vi "IdentifyAndReadInstr.vi"(8 "error in (no error)":errorcluster, 11 "VISA Resource Name":refnum<visa-resource-name>) -> (0 "error out":errorcluster, 1 "Instrument":T1=enum."LkShr 340 chA&B", 2 "Identified":bool, 3 "VISA Resource Name Out":refnum<visa-resource-name>)   [LabVIEW 2016]
uses:
  Device/Device type.ctl
  GPIB/VISA  Send Receive.vi
  <vilib>/Utility/error.llb/Error Cluster From Error Code.vi
  <vilib>/ErrorRing/Error Ring.xnode
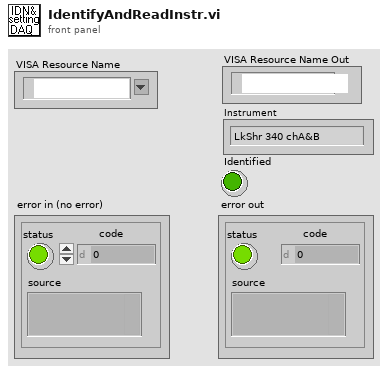
[diagram p1: front panel]
types:
  T1 = typedef "Device type.ctl" = enum16{"NONE", "Neocera 21", "LakeShore 335", "LakeShore 336", "LakeShore 340", "LkShr 340 chA&B", "LakeShore 370", "SRS 850", "SRS 830", "LR 700", "EG&G 5302", "EG&G 7260", "EG&G 7280", "AH 2500", "Keithley meter", "Keithley electrometer", "Keithley 182", "HP 5385", "HP 53181", "HP 53132", "ITC503", "IPS120", "Oxford Mercury IPS", "Oxford PS", "Test", "DC Facility Magnet", "Cryomagnetics PS", "Keithley 2400", "Keithley current source", "Cryo-Con 22C", "HP87NN", "HP4395A"}
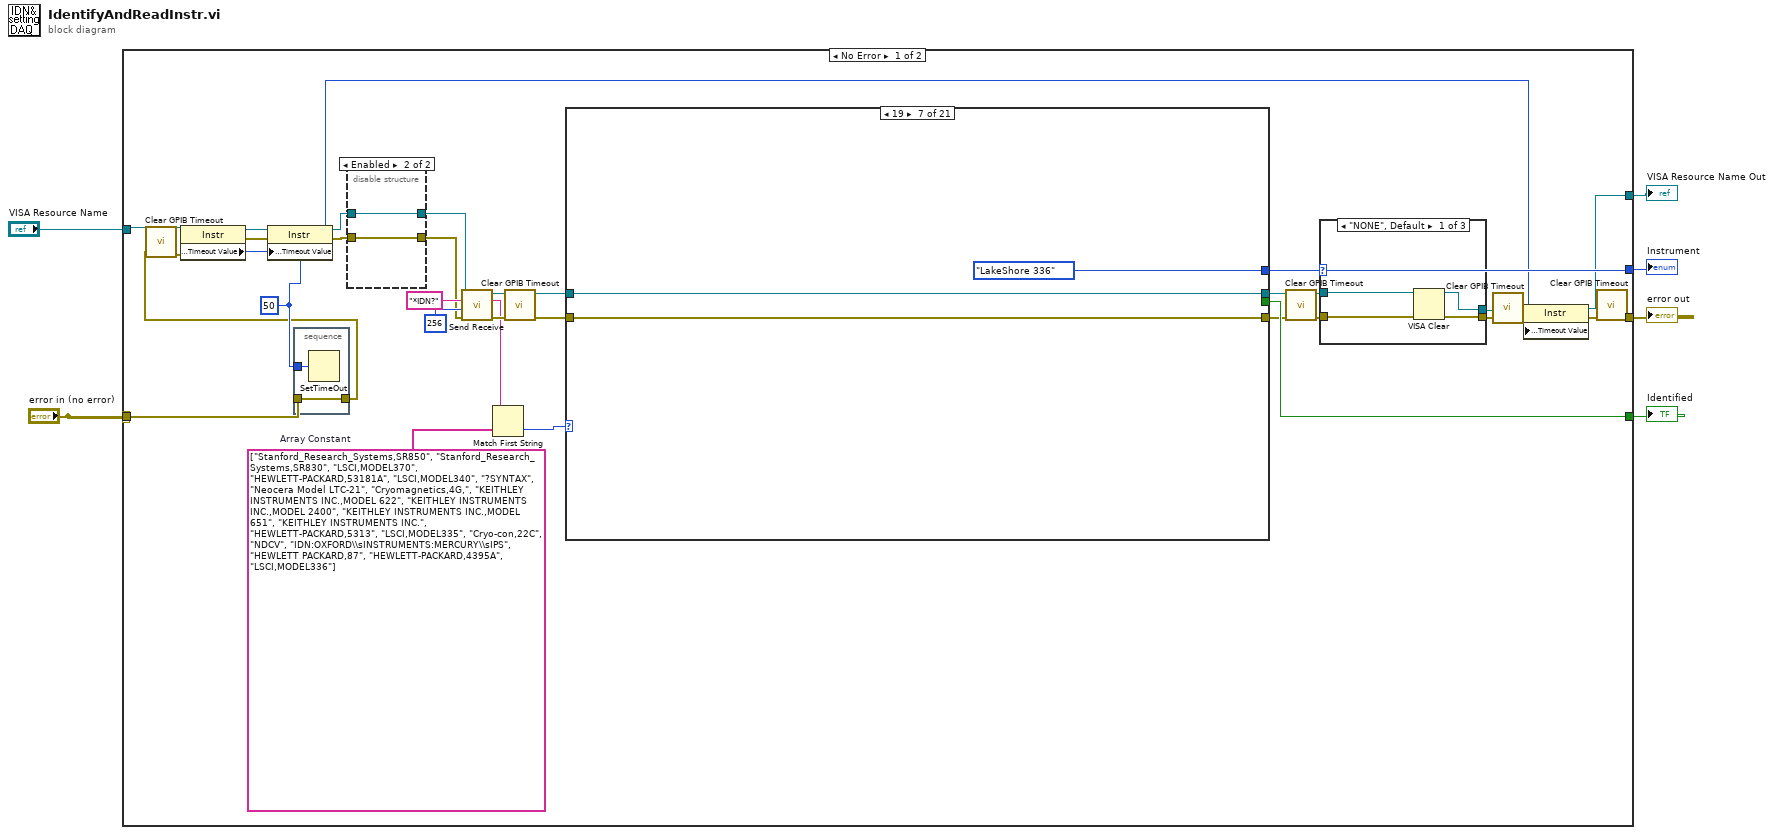
[diagram p0: block diagram]
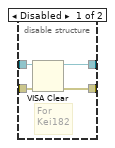
[diagram p2: hidden frame]
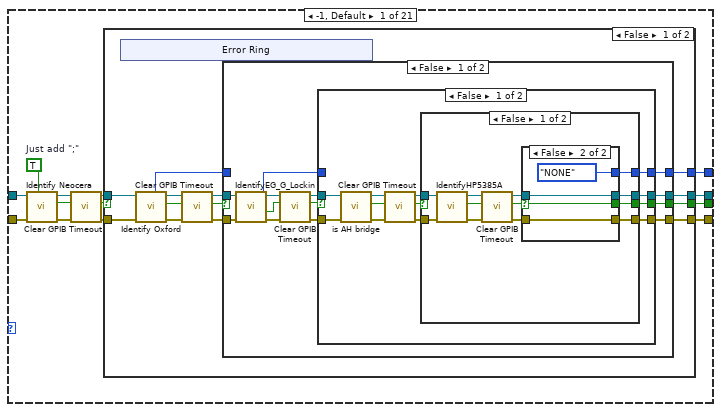
[diagram p5: hidden frame]
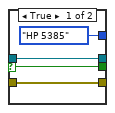
[diagram p6: hidden frame]
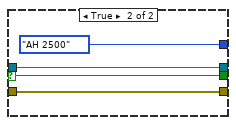
[diagram p7: hidden frame]
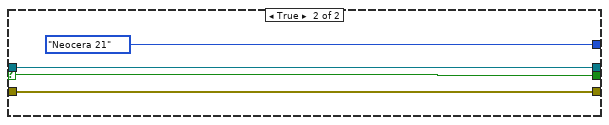
[diagram p10: hidden frame]
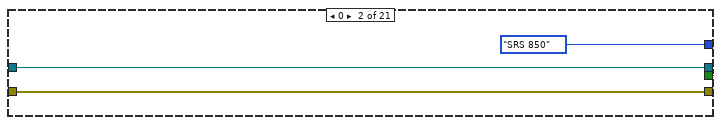
[diagram p11: hidden frame]
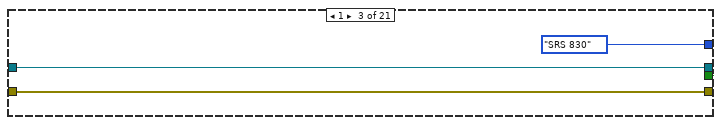
[diagram p12: hidden frame]
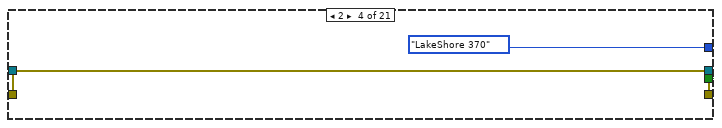
[diagram p13: hidden frame]
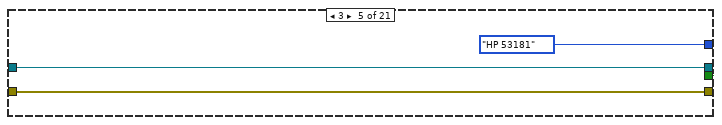
[diagram p14: hidden frame]
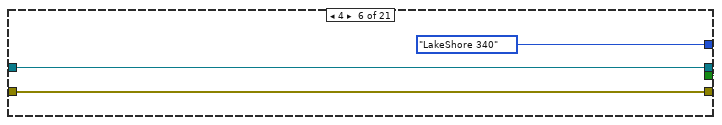
[diagram p15: hidden frame]
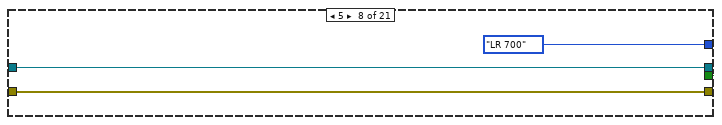
[diagram p16: hidden frame]
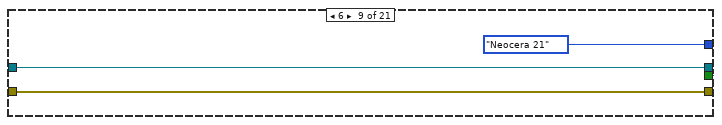
[diagram p17: hidden frame]
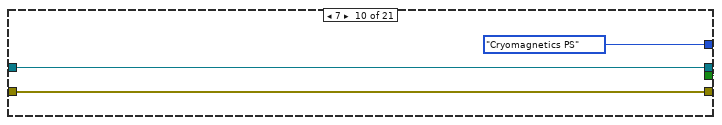
[diagram p18: hidden frame]
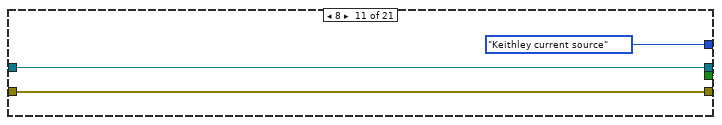
[diagram p19: hidden frame]
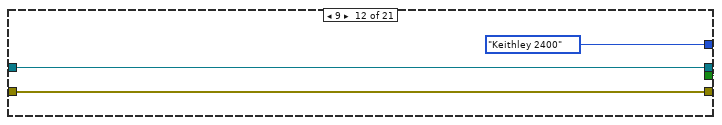
[diagram p20: hidden frame]
diagram:
  n1 = case shown="No Error" "error in (no error)" {
    tunnel: "error in (no error)" -> [w29 w230]
    tunnel: [w8 w230] -> w3
    tunnel: [w32 FALSE ("Identified")] -> w6
    tunnel: [w19 Device_type."NONE" ("Instrument")] -> w1
    tunnel: "VISA Resource Name" -> [w9 w228]
    tunnel: [w7 w228] -> w2
    frame No Error {
      w37 = string[] ["Stanford_Research_Systems,SR850", "Stanford_Research_Systems,SR830", "LSCI,MODEL370", "HEWLETT-PACKARD,53181A", "LSCI,MODEL340", "?SYNTAX", "Neocera Model LTC-21", "Cryomagnetics,4G,", "KEITHLEY INSTRUMENTS INC.,MODEL 622", "KEITHLEY INSTRUMENTS INC.,MODEL 2400", "KEITHLEY INSTRUMENTS INC.,MODEL 651", "KEITHLEY INSTRUMENTS INC.", "HEWLETT-PACKARD,5313", "LSCI,MODEL335", "Cryo-con,22C", "NDCV", "IDN:OXFORD\\sINSTRUMENTS:MERCURY\\sIPS", "HEWLETT PACKARD,87", "HEWLETT-PACKARD,4395A", "LSCI,MODEL336"]  # Array Constant
      w26 = 50 ("new timeout (10000)")
      n2 = stacked-sequence {
        tunnel: w29 -> [w53]
        tunnel: [w53] -> w10
        tunnel: w26 -> [w52]
        frame #0 {
          n3 = SetTimeOut(1:w52) -> ()  [unwired: 1 out]
        }
      }
      n4 = call "Clear GPIB Timeout.vi"("error in (no error)"=w10) -> ("error out"=w17:errorcluster)  [unwired: 1 in, 9 out]
      n5 = property class="Instr"(reference=w9, error in=w17) -> (reference out=w27:refnum<visa-resource-name>, error out=w25:errorcluster, "General Settings:Timeout Value"=w18:u32)
      n6 = property class="Instr"(reference=w27, error in=w25, "General Settings:Timeout Value"=w26) -> (reference out=w13:refnum<visa-resource-name>, error out=w14:errorcluster)
      n7 = disable-structure shown="Enabled" {
        disable-tunnel: w14 -> [w41 w42]
        disable-tunnel: w13 -> [w40 w43]
        disable-tunnel: [w39 w43] -> w12
        disable-tunnel: [w38 w42] -> w11
        frame Disabled {
          # "For\nKei182"
          n8 = VISA Clear(VISA resource name=w40, error in (no error)=w41) -> (VISA resource name out=w39:refnum<visa-resource-name>, error out=w38:errorcluster)
        }
        frame Enabled {
        }
      }
      n9 = call-poly "Send Receive.vi"("error in (no error)"=w11, "Receive count"=256 ("count"), "data string in"="*IDN?" ("data string"), "VISA Resource Name"=w12) -> ("error out"=w34:errorcluster, "data string out"=w33:string, "VISA Resource Name Out"=w28:refnum<visa-resource-name>)  [unwired: 5 in]
      n10 = Match First String(2:w37, 3:w33) -> (0:w36:i32)  [unwired: 1 out]
      n11 = call "Clear GPIB Timeout.vi"("error in (no error)"=w34) -> ("error out"=w31:errorcluster)  [unwired: 1 in, 9 out]
      n12 = case shown="19" w36 {
        tunnel: w31 -> [w63 w137 w141 w145 w149 w153 w157 w161 w165 w169 w173 w177 w183 w188 w192 w196 w200 w203 w215 w219 w223]
        tunnel: [w64 w137 w141 w145 w149 w153 w157 w161 w165 w169 w173 w177 w180 w188 w192 w196 w200 w202 w215 w219 w223] -> w24
        tunnel: [w61 TRUE ("Identified") TRUE ("Identified") TRUE ("Identified") TRUE ("Identified") TRUE ("Identified") TRUE ("Identified") TRUE ("Identified") TRUE ("Identified") TRUE ("Identified") TRUE ("Identified") TRUE ("Identified") TRUE ("Identified") TRUE ("Identified") TRUE ("Identified") TRUE ("Identified") TRUE ("Identified") TRUE ("Identified") TRUE ("Identified") TRUE ("Identified") TRUE ("Identified")] -> w32
        tunnel: [w62 Device_type."SRS 850" ("Instrument") Device_type."SRS 830" ("Instrument") Device_type."LakeShore 370" ("Instrument") Device_type."HP 53181" ("Instrument") Device_type."LakeShore 340" ("Instrument") Device_type."LakeShore 336" ("Instrument") Device_type."LR 700" ("Instrument") Device_type."Neocera 21" ("Instrument") Device_type."Cryomagnetics PS" ("Instrument") Device_type."Keithley current source" ("Instrument") Device_type."Keithley 2400" ("Instrument") Device_type."Keithley electrometer" ("Instrument") Device_type."Keithley meter" ("Instrument") Device_type."HP 53132" ("Instrument") Device_type."LakeShore 335" ("Instrument") Device_type."Cryo-Con 22C" ("Instrument") Device_type."Keithley 182" ("Instrument") Device_type."Oxford Mercury IPS" ("Instrument") Device_type."HP87NN" ("Instrument") Device_type."HP4395A" ("Instrument")] -> w19
        tunnel: w28 -> [w59 w136 w140 w144 w148 w152 w156 w160 w164 w168 w172 w176 w182 w187 w191 w195 w199 w206 w216 w220 w224]
        tunnel: [w60 w136 w140 w144 w148 w152 w156 w160 w164 w168 w172 w176 w179 w187 w191 w195 w199 w204 w216 w220 w224] -> w22
        frame -1, Default {
          w55 = TRUE  # Just add ";"
          n13 = call "Identify Neocera.vi"("Just add \";\""=w55, "error in (no error)"=w63, "VISA Resource Name"=w59) -> ("error out"=w57:errorcluster, "Identified"=w54:bool, "VISA Resource Name Out"=w58:refnum<visa-resource-name>)  [unwired: 6 out]
          n14 = call "Clear GPIB Timeout.vi"("error in (no error)"=w57) -> ("error out"=w56:errorcluster)  [unwired: 1 in, 9 out]
          n15 = case shown="False" w54 {
            selector: w54 -> [_ w132]
            tunnel: [w75 w133] -> w64
            tunnel: [w74 Device_type."Neocera 21" ("Instrument")] -> w62
            tunnel: [w73 w132] -> w61
            tunnel: [w72 w131] -> w60
            tunnel: w58 -> [w68 w131]
            tunnel: w56 -> [w70 w133]
            frame False {
              n16 = xnode "Error Ring"() -> ()  [unwired: 1 out]
              n17 = call "Identify Oxford.vi"("error in (no error)"=w70, "VISA resource name"=w68) -> ("error out"=w69:errorcluster, "It's from Oxford!"=w66:bool, "VISA resource name out"=w67:refnum<visa-resource-name>, "Instrument"=w65:T1)  [unwired: 5 in, 1 out]
              n18 = call "Clear GPIB Timeout.vi"("error in (no error)"=w69) -> ("error out"=w71:errorcluster)  [unwired: 1 in, 9 out]
              n19 = case shown="False" w66 {
                selector: w66 -> [_ w128]
                tunnel: [w90 w129] -> w75
                tunnel: w71 -> [w89 w129]
                tunnel: [w87 w127] -> w74
                tunnel: [w86 w128] -> w73
                tunnel: w67 -> [w82 w130]
                tunnel: [w80 w130] -> w72
                tunnel: w65 -> [_ w127]
                frame False {
                  n20 = call "IdentifyEG_G_Lockin.vi"("error in (no error)"=w89, "VISA Resource Name"=w82) -> ("error out"=w88:errorcluster, "Identified"=w83:bool, "Instrument"=w85:T1, "VISA Resource Name Out"=w81:refnum<visa-resource-name>)  [unwired: 6 out]
                  n21 = call "Clear GPIB Timeout.vi"("error in (no error)"=w88) -> ("error out"=w84:errorcluster)  [unwired: 1 in, 9 out]
                  n22 = case shown="False" w83 {
                    selector: w83 -> [_ w123]
                    tunnel: [w96 w126] -> w90
                    tunnel: w84 -> [w100 w126]
                    tunnel: [w94 w125] -> w87
                    tunnel: [w99 w123] -> w86
                    tunnel: w85 -> [_ w125]
                    tunnel: w81 -> [w93 w124]
                    tunnel: [w91 w124] -> w80
                    frame False {
                      n23 = call "is AH bridge.vi"("error in (no error)"=w100, "VISA Resource Name"=w93) -> ("error out"=w97:errorcluster, "is AH?"=w98:bool, "VISA Resource Name Out"=w92:refnum<visa-resource-name>)  [unwired: 7 out]
                      n24 = call "Clear GPIB Timeout.vi"("error in (no error)"=w97) -> ("error out"=w95:errorcluster)  [unwired: 1 in, 9 out]
                      n25 = case shown="False" w98 {
                        selector: w98 -> [_ w119]
                        tunnel: [w109 Device_type."AH 2500" ("Instrument")] -> w94
                        tunnel: [w101 w119] -> w99
                        tunnel: w95 -> [w110 w122]
                        tunnel: [w103 w122] -> w96
                        tunnel: w92 -> [w108 w121]
                        tunnel: [w102 w121] -> w91
                        frame False {
                          n26 = call "IdentifyHP5385A.vi"("error in (no error)"=w110, "VISA Resource Name"=w108) -> ("error out"=w105:errorcluster, "Identified"=w107:bool, "VISA Resource Name Out"=w106:refnum<visa-resource-name>)  [unwired: 7 out]
                          n27 = call "Clear GPIB Timeout.vi"("error in (no error)"=w105) -> ("error out"=w104:errorcluster)  [unwired: 1 in, 9 out]
                          n28 = case shown="False" w107 {
                            selector: w107 -> [w111 w115]
                            tunnel: [Device_type."HP 5385" ("Instrument") Device_type."NONE" ("Instrument")] -> w109
                            tunnel: w104 -> [w112 w116]
                            tunnel: w106 -> [w113 w117]
                            tunnel: [w112 w116] -> w103
                            tunnel: [w113 w117] -> w102
                            tunnel: [w111 w115] -> w101
                            frame True {
                            }
                            frame False {
                            }
                          }
                        }
                        frame True {
                        }
                      }
                    }
                    frame True {
                    }
                  }
                }
                frame True {
                }
              }
            }
            frame True {
            }
          }
        }
        frame 0 {
        }
        frame 1 {
        }
        frame 2 {
        }
        frame 3 {
        }
        frame 4 {
        }
        frame 19 {
        }
        frame 5 {
        }
        frame 6 {
        }
        frame 7 {
        }
        frame 8 {
        }
        frame 9 {
        }
        frame 10 {
          n29 = VISA Write(VISA resource name=w182, write buffer=":INIT", error in (no error)=w183) -> (VISA resource name out=w179:refnum<visa-resource-name>, error out=w180:errorcluster)  [unwired: 1 out]
        }
        frame 11 {
        }
        frame 12 {
        }
        frame 13 {
        }
        frame 14 {
        }
        frame 15 {
          n30 = disable-structure shown="Disabled" {
            disable-tunnel: w206 -> [w212 w214]
            disable-tunnel: [w211 w214] -> w204
            disable-tunnel: w203 -> [w210 w213]
            disable-tunnel: [w209 w213] -> w202
            frame Disabled {
              # "Skip prefix in returnet data"
              n31 = VISA Write(VISA resource name=w212, write buffer="G0", error in (no error)=w210) -> (VISA resource name out=w211:refnum<visa-resource-name>, error out=w209:errorcluster)  [unwired: 1 out]
            }
            frame Enabled {
            }
          }
        }
        frame 16 {
        }
        frame 17 {
        }
        frame 18 {
        }
      }
      n32 = call "Clear GPIB Timeout.vi"("error in (no error)"=w24) -> ("error out"=w23:errorcluster)  [unwired: 1 in, 9 out]
      n33 = case shown="\"NONE\", Default" w19 {
        tunnel: w23 -> [w47 w49 w51]
        tunnel: w22 -> [w46 w48 w50]
        tunnel: [w45 w49 w51] -> w16
        tunnel: [w44 w48 w50] -> w20
        frame "NONE", Default {
          n34 = VISA Clear(VISA resource name=w46, error in (no error)=w47) -> (VISA resource name out=w44:refnum<visa-resource-name>, error out=w45:errorcluster)
        }
        frame "Keithley electrometer" {
        }
        frame "Keithley 182" {
        }
      }
      n35 = call "Clear GPIB Timeout.vi"("error in (no error)"=w16) -> ("error out"=w15:errorcluster)  [unwired: 1 in, 9 out]
      n36 = property class="Instr"(reference=w20, error in=w15, "General Settings:Timeout Value"=w18) -> (reference out=w7:refnum<visa-resource-name>, error out=w21:errorcluster)
      n37 = call "Clear GPIB Timeout.vi"("error in (no error)"=w21) -> ("error out"=w8:errorcluster)  [unwired: 10 in]
    }
    frame Error {
    }
  }
  "error out" <- w3
  "Identified" <- w6
  "Instrument" <- w1
  "VISA Resource Name Out" <- w2
